vi "Reorder Connector Pane Object Refs.vi"(8 "Error In":errorcluster, 10 "Connector Pane Patter":u32, 11 "Connector Pane Object Refs":refnum<vi>[](array[refnum])) -> (0 "Error Out":errorcluster, 3 "Connector Pane Object Refs":refnum<vi>[][](array[refnum]))   [LabVIEW 2011, in "LVH-Toolbox.lvlib"]
uses:
  <vilib>/LabVIEW Hacker/LVH-Toolbox/LVH-Toolbox.lvlib
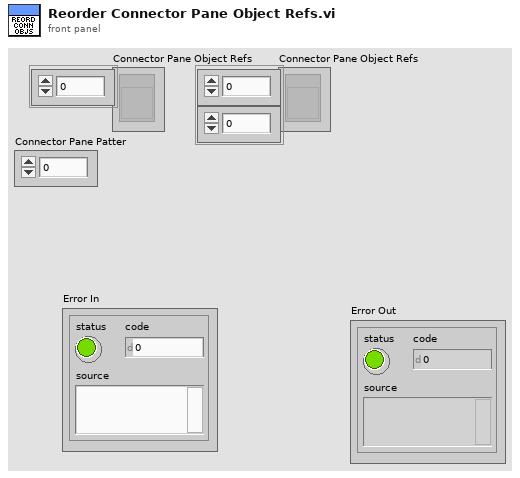
[diagram p1: front panel]
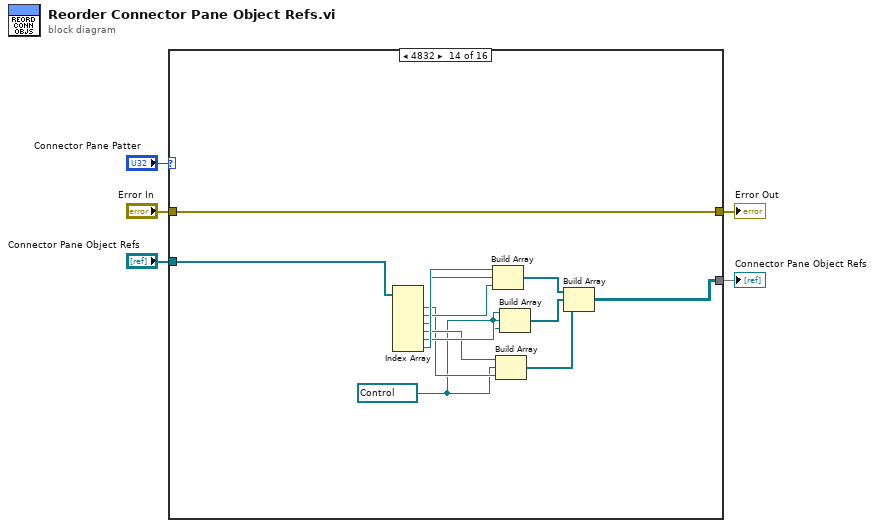
[diagram p0: block diagram]
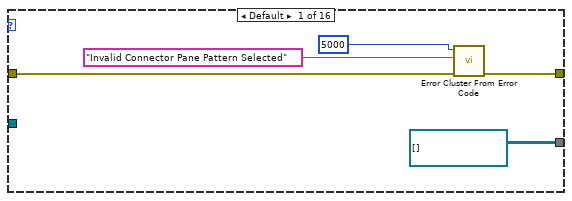
[diagram p2: hidden frame]
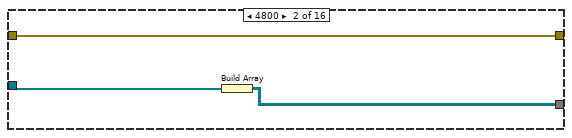
[diagram p3: hidden frame]
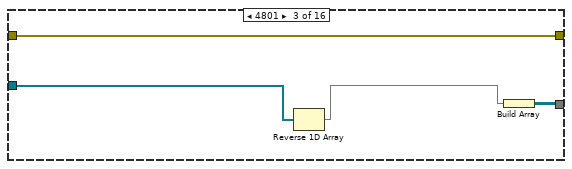
[diagram p4: hidden frame]
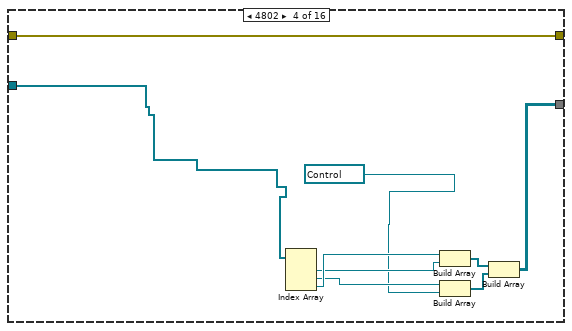
[diagram p5: hidden frame]
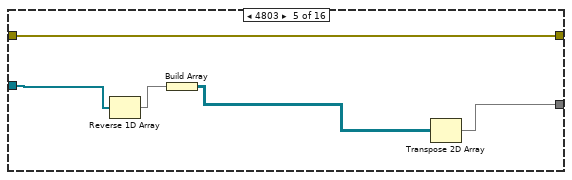
[diagram p6: hidden frame]
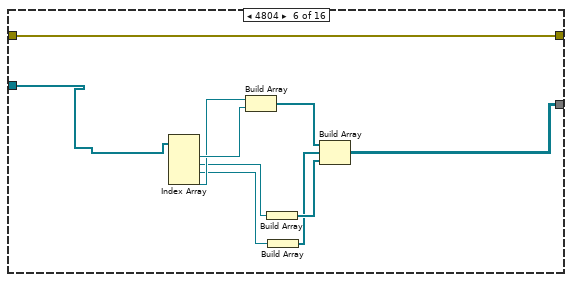
[diagram p7: hidden frame]
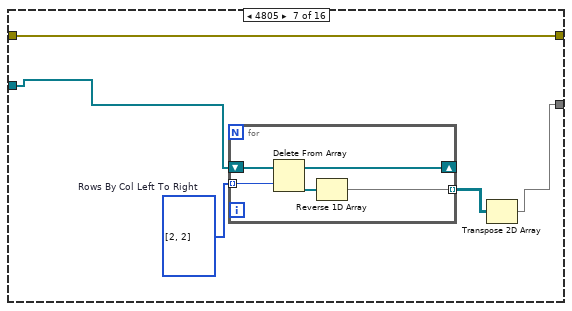
[diagram p8: hidden frame]
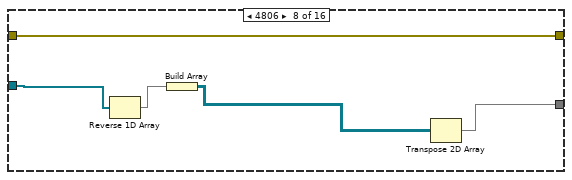
[diagram p9: hidden frame]
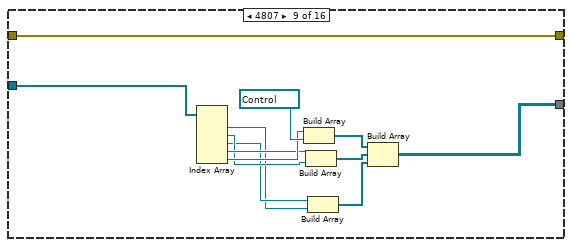
[diagram p10: hidden frame]
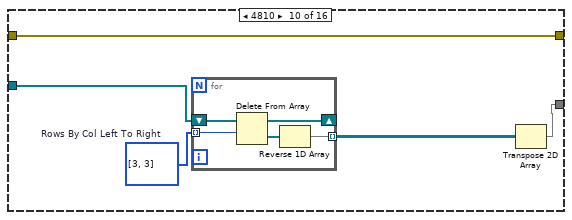
[diagram p11: hidden frame]
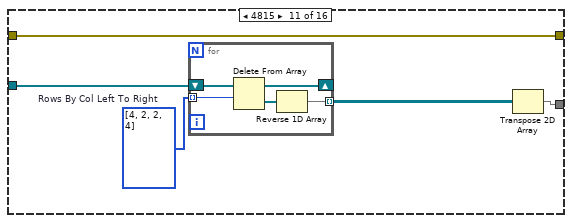
[diagram p12: hidden frame]
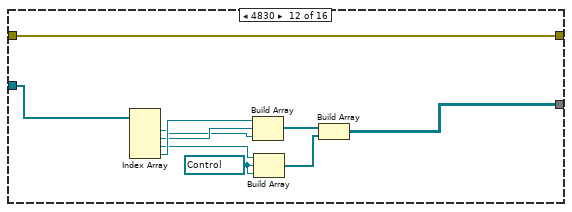
[diagram p13: hidden frame]
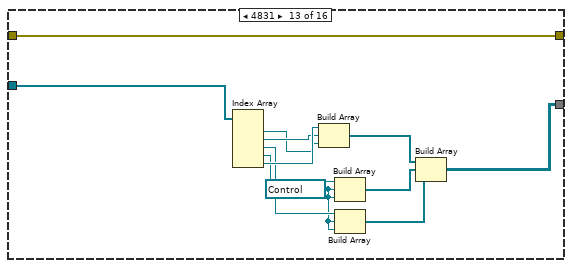
[diagram p14: hidden frame]
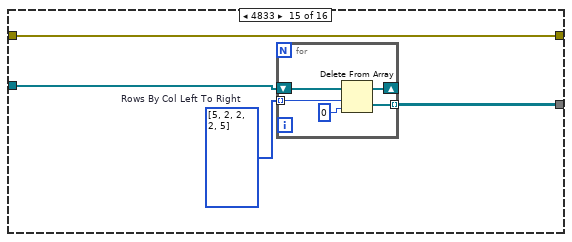
[diagram p15: hidden frame]
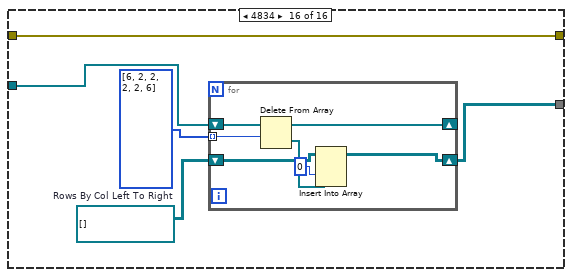
[diagram p16: hidden frame]
diagram:
  n1 = case shown="4832" "Connector Pane Patter" {
    tunnel: [w10 w11 w17 w26 w31 w41 w46 w56 w68 w73 w83 w98 w110 w123 w127 w137] -> w5
    tunnel: "Error In" -> [w7 w11 w17 w26 w31 w41 w46 w56 w68 w73 w83 w98 w110 w123 w127 w137]
    tunnel: "Connector Pane Object Refs" -> [_ w13 w15 w25 w28 w40 w44 w53 w67 w70 w81 w97 w109 w122 w125 w136]
    tunnel: [refnum<vi>[][] [] ("Connector Pane Object Refs") w12 w16 w18 w29 w35 w43 w54 w57 w69 w79 w90 w99 w121 w124 w133] -> w2
    frame Default {
      n2 = call <vilib>:"Error Cluster From Error Code.vi"("error in (no error)"=w7, "error message (\"\")"="Invalid Connector Pane Pattern Selected" ("error message (\"\")"), "error code (0)"=5000) -> ("error out"=w10:errorcluster)  [unwired: 6 in]
    }
    frame 4800 {
      n3 = Build Array(w13) -> (w12:refnum<vi>[][])
    }
    frame 4801 {
      n4 = Reverse 1D Array(array=w15) -> (reversed array=w14:refnum<vi>[])
      n5 = Build Array(w14) -> (w16:refnum<vi>[][])
    }
    frame 4802 {
      n6 = Index Array(array=w25) -> (element #1=w23:refnum<vi>, element #2=w22:refnum<vi>, element #3=w24:refnum<vi>)  [unwired: 3 in]
      n7 = Build Array(w24, w23) -> (w20:refnum<vi>[])
      n8 = Build Array(w22, refnum<vi> refnum ("element")) -> (w19:refnum<vi>[])
      n9 = Build Array(w20, w19) -> (w18:refnum<vi>[][])
    }
    frame 4803 {
      n10 = Reverse 1D Array(array=w28) -> (reversed array=w27:refnum<vi>[])
      n11 = Build Array(w27) -> (w30:refnum<vi>[][])
      n12 = Transpose 2D Array(2D array=w30) -> (transposed array=w29:refnum<vi>[][])
    }
    frame 4804 {
      n13 = Index Array(array=w40) -> (element #1=w39:refnum<vi>, element #2=w37:refnum<vi>, element #3=w34:refnum<vi>, element #4=w38:refnum<vi>)  [unwired: 4 in]
      n14 = Build Array(w38, w39) -> (w36:refnum<vi>[])
      n15 = Build Array(w37) -> (w33:refnum<vi>[])
      n16 = Build Array(w34) -> (w32:refnum<vi>[])
      n17 = Build Array(w36, w32, w33) -> (w35:refnum<vi>[][])
    }
    frame 4805 {
      w45 = i32[] [2, 2]  # Rows By Col Left To Right
      n18 = for {
        tunnel: [w50] -> w42 mode=indexing
        shift-right: [w51] -> _
        shift-left: w44 -> [w49]
        tunnel: w45 -> [w47] mode=indexing
        n19 = Delete From Array(array=w49, length=w47) -> (deleted portion=w48:refnum<vi>[], array with subset deleted=w51:refnum<vi>[])  [unwired: 1 in]
        n20 = Reverse 1D Array(array=w48) -> (reversed array=w50:refnum<vi>[])
      }
      n21 = Transpose 2D Array(2D array=w42) -> (transposed array=w43:refnum<vi>[][])
    }
    frame 4806 {
      n22 = Reverse 1D Array(array=w53) -> (reversed array=w52:refnum<vi>[])
      n23 = Build Array(w52) -> (w55:refnum<vi>[][])
      n24 = Transpose 2D Array(2D array=w55) -> (transposed array=w54:refnum<vi>[][])
    }
    frame 4807 {
      n25 = Index Array(array=w67) -> (element #1=w61:refnum<vi>, element #2=w63:refnum<vi>, element #3=w62:refnum<vi>, element #4=w64:refnum<vi>, element #5=w65:refnum<vi>)  [unwired: 5 in]
      n26 = Build Array(w65, refnum<vi> refnum ("element")) -> (w60:refnum<vi>[])
      n27 = Build Array(w64, w63) -> (w59:refnum<vi>[])
      n28 = Build Array(w62, w61) -> (w58:refnum<vi>[])
      n29 = Build Array(w60, w59, w58) -> (w57:refnum<vi>[][])
    }
    frame 4810 {
      w71 = i32[] [3, 3]  # Rows By Col Left To Right
      n30 = for {
        tunnel: [w77] -> w72 mode=indexing
        shift-right: [w78] -> _
        shift-left: w70 -> [w76]
        tunnel: w71 -> [w74] mode=indexing
        n31 = Delete From Array(array=w76, length=w74) -> (deleted portion=w75:refnum<vi>[], array with subset deleted=w78:refnum<vi>[])  [unwired: 1 in]
        n32 = Reverse 1D Array(array=w75) -> (reversed array=w77:refnum<vi>[])
      }
      n33 = Transpose 2D Array(2D array=w72) -> (transposed array=w69:refnum<vi>[][])
    }
    frame 4815 {
      w80 = i32[] [4, 2, 2, 4]  # Rows By Col Left To Right
      n34 = for {
        tunnel: [w87] -> w82 mode=indexing
        shift-right: [w88] -> _
        shift-left: w81 -> [w86]
        tunnel: w80 -> [w84] mode=indexing
        n35 = Delete From Array(array=w86, length=w84) -> (deleted portion=w85:refnum<vi>[], array with subset deleted=w88:refnum<vi>[])  [unwired: 1 in]
        n36 = Reverse 1D Array(array=w85) -> (reversed array=w87:refnum<vi>[])
      }
      n37 = Transpose 2D Array(2D array=w82) -> (transposed array=w79:refnum<vi>[][])
    }
    frame 4830 {
      w89 = refnum<vi> refnum ("element")
      n38 = Index Array(array=w97) -> (element #1=w94:refnum<vi>, element #2=w95:refnum<vi>, element #3=w93:refnum<vi>, element #4=w96:refnum<vi>)  [unwired: 4 in]
      n39 = Build Array(w96, w95, w94) -> (w92:refnum<vi>[])
      n40 = Build Array(w93, w89, w89) -> (w91:refnum<vi>[])
      n41 = Build Array(w92, w91) -> (w90:refnum<vi>[][])
    }
    frame 4831 {
      w103 = refnum<vi> refnum ("element")
      n42 = Index Array(array=w109) -> (element #1=w105:refnum<vi>, element #2=w106:refnum<vi>, element #3=w104:refnum<vi>, element #4=w107:refnum<vi>, element #5=w108:refnum<vi>)  [unwired: 5 in]
      n43 = Build Array(w108, w106, w105) -> (w102:refnum<vi>[])
      n44 = Build Array(w107, w103, w103) -> (w101:refnum<vi>[])
      n45 = Build Array(w104, w103, w103) -> (w100:refnum<vi>[])
      n46 = Build Array(w102, w101, w100) -> (w99:refnum<vi>[][])
    }
    frame 4832 {
      w114 = refnum<vi> refnum ("element")
      n47 = Index Array(array=w122) -> (element #1=w115:refnum<vi>, element #2=w118:refnum<vi>, element #3=w119:refnum<vi>, element #4=w116:refnum<vi>, element #5=w117:refnum<vi>, element #6=w120:refnum<vi>)  [unwired: 6 in]
      n48 = Build Array(w120, w119, w118) -> (w113:refnum<vi>[])
      n49 = Build Array(w116, w114, w115) -> (w111:refnum<vi>[])
      n50 = Build Array(w117, w114, w114) -> (w112:refnum<vi>[])
      n51 = Build Array(w113, w112, w111) -> (w121:refnum<vi>[][])
    }
    frame 4833 {
      w126 = i32[] [5, 2, 2, 2, 5]  # Rows By Col Left To Right
      n52 = for {
        tunnel: w126 -> [w131] mode=indexing
        tunnel: [w129] -> w124 mode=indexing
        shift-right: [w130] -> _
        shift-left: w125 -> [w132]
        n53 = Delete From Array(array=w132, length=w131, index=0) -> (deleted portion=w129:refnum<vi>[], array with subset deleted=w130:refnum<vi>[])
      }
    }
    frame 4834 {
      w135 = i32[] [6, 2, 2, 2, 2, 6]  # Rows By Col Left To Right
      n54 = for {
        shift-right: [w144] -> _
        shift-left: w136 -> [w143]
        tunnel: w135 -> [w142] mode=indexing
        shift-right: [w140] -> w133
        shift-left: refnum<vi>[][] [] ("array") -> [w141]
        n55 = Delete From Array(array=w143, length=w142) -> (deleted portion=w139:refnum<vi>[], array with subset deleted=w144:refnum<vi>[])  [unwired: 1 in]
        n56 = Insert Into Array(array=w141, index (col)=0 ("index (row)"), new element=w139) -> (w140:refnum<vi>[][])  [unwired: 1 in]
      }
    }
  }
  "Error Out" <- w5
  "Connector Pane Object Refs" <- w2
